vi "Read Linker Info from File.vi"(8 "error in (no error)":errorcluster, 9 "polys & tds":bool, 10 "recursive?":bool, 11 "paths to read":path[](array[path])) -> (0 "error out":errorcluster, 2 "Read Linker Info from File":T1(array[cluster]))   [LabVIEW 2020, in "Save for Previous Version.lvlib"]
uses:
  Save for Previous Version.lvlib
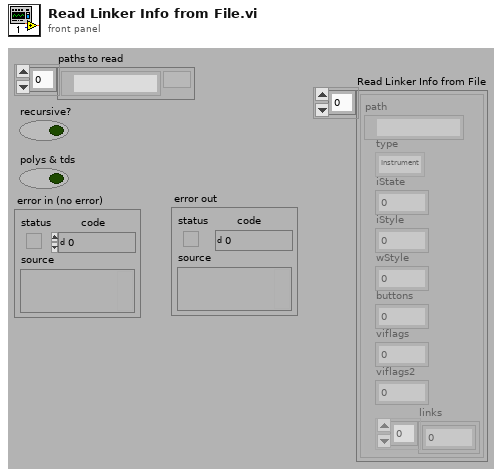
[diagram p1: front panel]
types:
  T1 = cluster{"path":path, "type":enum32{"Instrument", "Control", "CIN", "External subroutine", "Shared library", "Run-time menu", "Help file", "Palette menu"}, "iState":u32, "iStyle":u16, "wStyle":u16, "buttons":u16, "viflags":u32, "viflags2":u32, "links":u32[]}[]
  T2 = cluster{"path":path, "type":enum32{"Instrument", "Control", "CIN", "External subroutine", "Shared library", "Run-time menu", "Help file", "Palette menu", "Polymorphic VI", "Library"}, "iState":u32, "iStyle":u16, "wStyle":u16, "buttons":u16, "viflags":u32, "viflags2":u32, "links":u32[]}[]
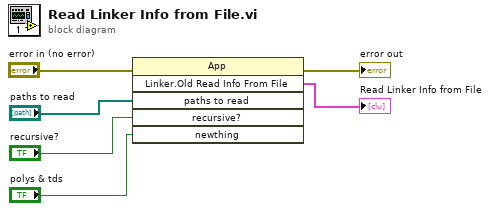
[diagram p0: block diagram]
diagram:
  n1 = invoke class="App" method="Linker.Old Read Info From File"(error in="error in (no error)", "paths to read"="paths to read", "recursive?"="recursive?", "newthing"="polys & tds") -> (error out=→"error out":errorcluster, "Read Linker Info from File"=→"Read Linker Info from File":T2)  [unwired: 2 in, 4 out]
